vi "Max Search.vi"() -> ()   [LabVIEW 2021]
panel:
  out "Iteration Count":dbl
  out "Max":dbl
  in  "Number of Iterations":i32
  out "Random Number":dbl
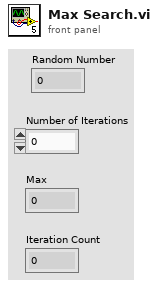
[diagram p1: front panel]
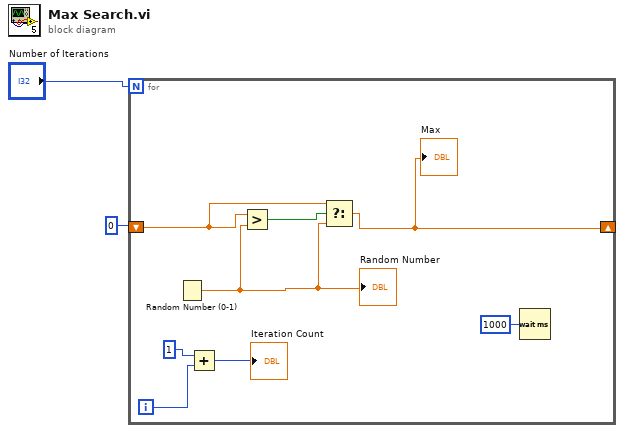
[diagram p0: block diagram]
diagram:
  n1 = for {
    N: "Number of Iterations" -> [_]
    shift-right: [w6] -> _
    shift-left: 0 -> [w7]
    i -> [w4]
    n2 = Random Number (0-1)() -> (number: 0 to 1=w9:dbl)
    "Random Number" <- w9
    n3 = Add(x=1, y=w4) -> (x+y=→"Iteration Count":i32)
    n4 = Greater?(x=w7, y=w9) -> (0:w8:bool)
    n5 = Select(t=w7, s=w8, f=w9) -> (s? t:f=w6:dbl)
    "Max" <- w6
    n6 = Wait (ms)(milliseconds to wait=u32 1000) -> ()  [unwired: 1 out]
  }
